vi "mk.vi"() -> ()   [LabVIEW 2016]
uses:
  <vilib>/Utility/file.llb/Write Delimited Spreadsheet (DBL).vi
panel:
  in  "Boolean 2":bool
  out "midiendo histeresis":bool
  in  "Boolean":bool
  in  "Lecturas":i32=5 min=1
  out "upset multimetro":dbl
  out "upset lockin":dbl
  out "division":cluster{"array":dbl[], "array":dbl[]}(graph)
  out "multimetro":cluster{"array":dbl[], "array":dbl[]}(graph)
  in  "Nombre (guardar como .txt)":path
  out "campo":dbl
  in  "paso":dbl
  in  "final":dbl
  in  "inicio":dbl
  out "Lock_In":cluster{"array":dbl[], "array":dbl[]}(graph)
  # "normal"
  # "histeresis"
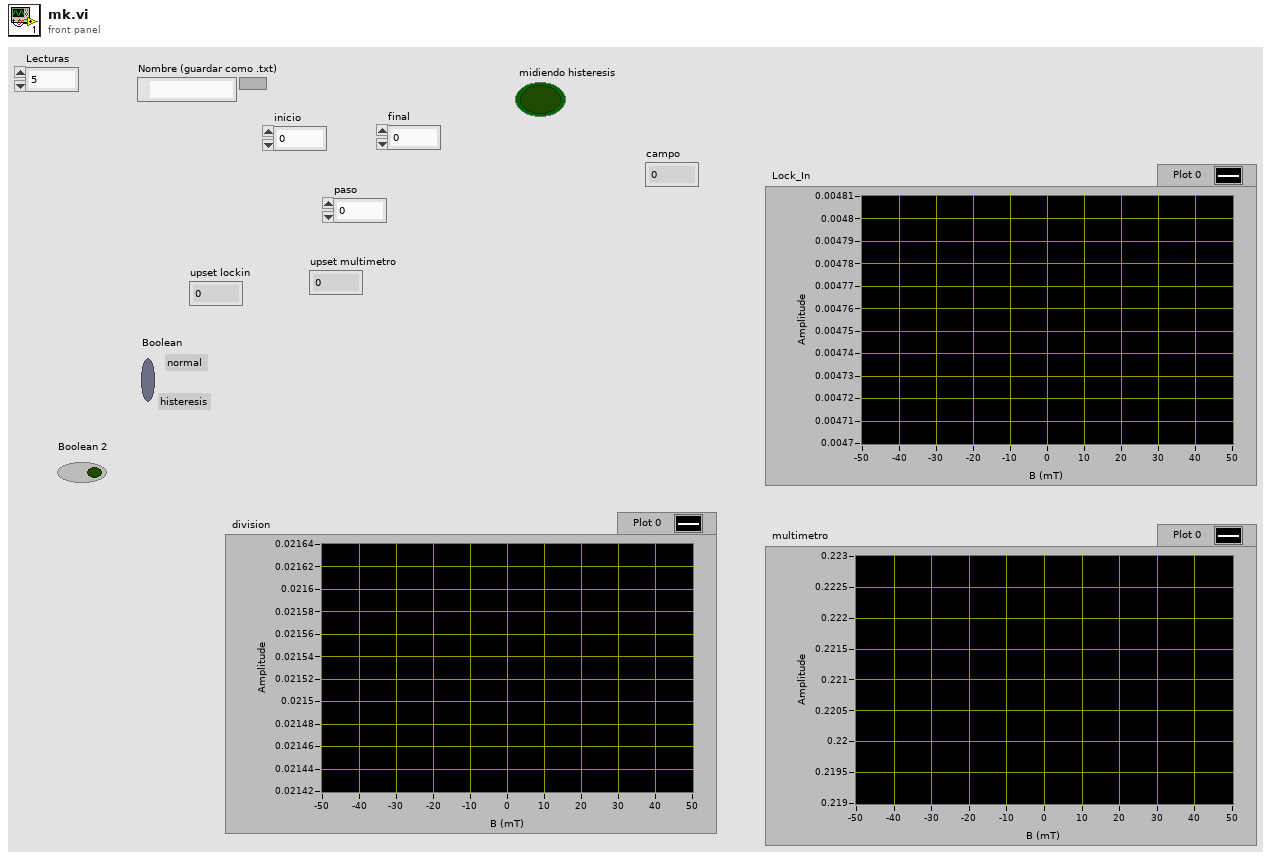
[diagram p1: front panel]
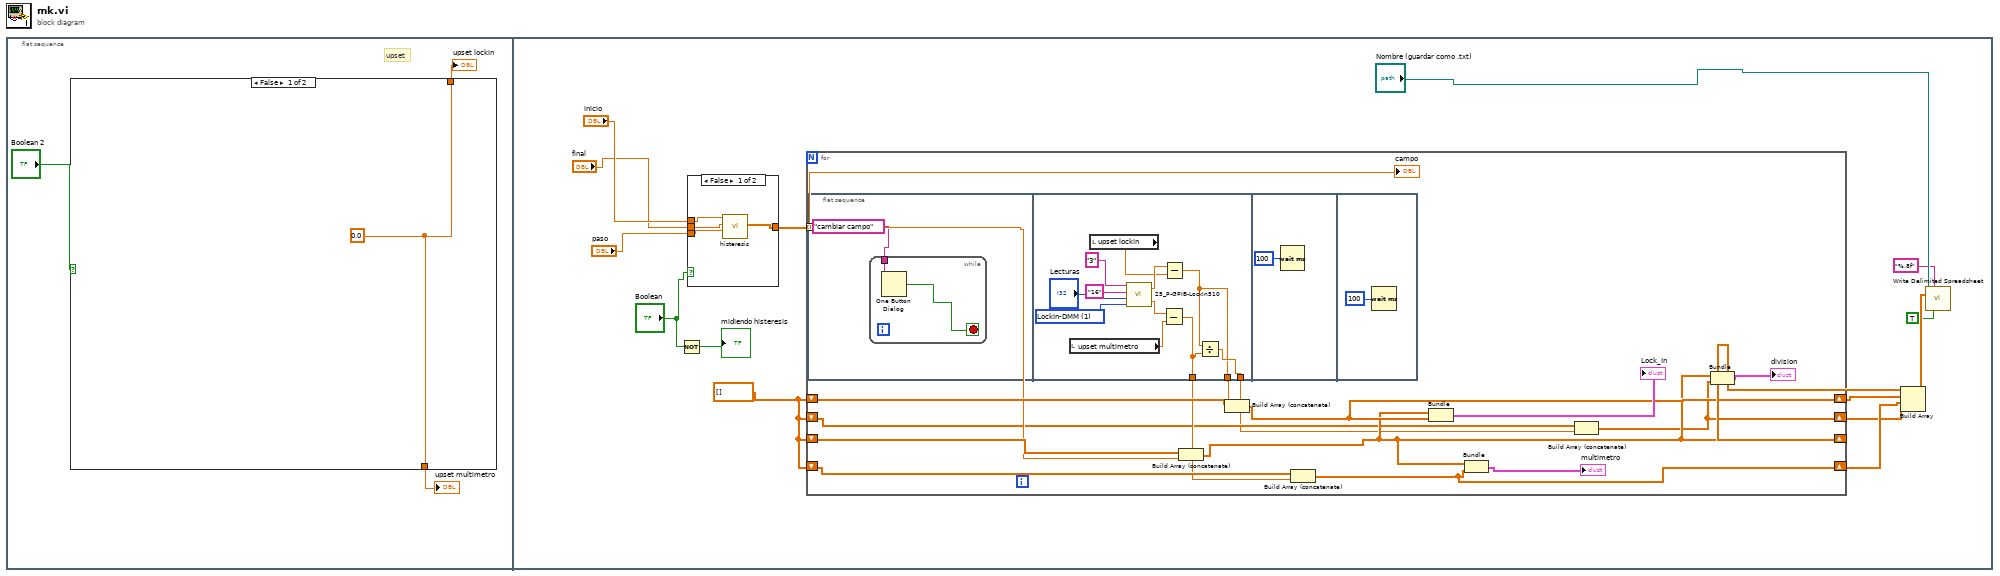
[diagram p0: block diagram]
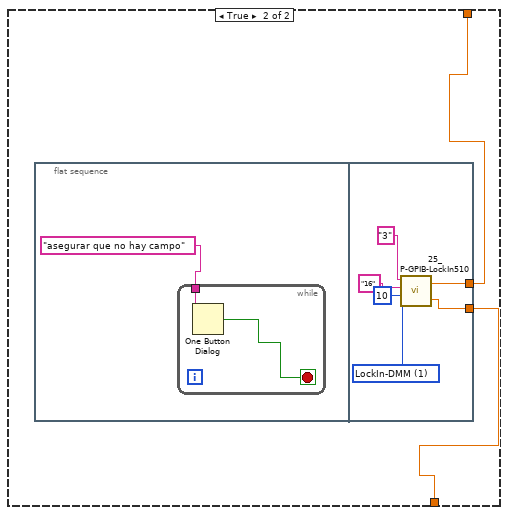
[diagram p2: hidden frame]
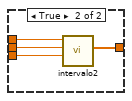
[diagram p3: hidden frame]
diagram:
  n1 = flat-sequence {
    frame #0 {
      # "upset"
      n2 = case shown="False" "Boolean 2" {
        tunnel: [w4 w6] -> w2
        tunnel: [w4 w5] -> w1
        frame False {
          w4 = 0.0
        }
        frame True {
          n3 = flat-sequence {
            tunnel: [w12] -> w6
            tunnel: [w11] -> w5
            frame #0 {
              n4 = while {
                tunnel: "asegurar que no hay campo" ("message") -> [w8]
                stop <- w9 stop-if-true
                n5 = One Button Dialog(message=w8) -> (true=w9:bool)  [unwired: 1 in]
              }
            }
            frame #1 {
              w13 = u16 1 items=["LockIn", "LockIn-DMM"] ("Tipo")
              n6 = call "25_P-GPIB-LockIn510.vi"("Tipo"=w13, "Lecturas"=10, "P-DMM"="16", "P-LockIn"="3") -> ("DMM"=w11:dbl, "LockIn"=w12:dbl)
            }
          }
        }
      }
      "upset lockin" <- w2
      "upset multimetro" <- w1
    }
    frame #1 {
      w19 = dbl[] []
      n7 = Not(x="Boolean") -> (.not. x?=→"midiendo histeresis":bool)
      n8 = case shown="False" "Boolean" {
        tunnel: "inicio" -> [w33 w38]
        tunnel: "final" -> [w32 w37]
        tunnel: "paso" -> [w31 w36]
        tunnel: [w34 w35] -> w27
        frame False {
          n9 = call "histeresis.vi"("paso"=w31, "fin"=w32, "inicio"=w33) -> ("Array"=w34:dbl[])  [unwired: 8 in]
        }
        frame True {
          n10 = call "intervalo2.vi"("incremento"=w36, "fin"=w37, "inicio"=w38) -> ("Array"=w35:dbl[])  [unwired: 8 in]
        }
      }
      n11 = for {
        tunnel: w27 -> [w49] mode=indexing
        shift-right: [w47] -> w21
        shift-left: w19 -> [w52]
        shift-right: [w43] -> w25
        shift-left: w19 -> [w51]
        shift-right: [w45] -> w20
        shift-left: w19 -> [w46]
        shift-right: [w39] -> w18
        shift-left: w19 -> [w41]
        n12 = flat-sequence {
          tunnel: [w62] -> w53
          tunnel: [w59] -> w42
          tunnel: [w63] -> w40
          frame #0 {
            n13 = while {
              tunnel: "cambiar campo" ("message") -> [w55]
              stop <- w56 stop-if-true
              n14 = One Button Dialog(message=w55) -> (true=w56:bool)  [unwired: 1 in]
            }
          }
          frame #1 {
            w64 = u16 1 items=["LockIn", "LockIn-DMM"] ("Tipo")
            n15 = local read "upset multimetro"() -> (w57:dbl)
            n16 = local read "upset lockin"() -> (w60:dbl)
            n17 = call "25_P-GPIB-LockIn510.vi"("Tipo"=w64, "Lecturas"="Lecturas", "P-DMM"="16", "P-LockIn"="3") -> ("DMM"=w58:dbl, "LockIn"=w61:dbl)
            n18 = Subtract(x=w58, y=w57) -> (x-y=w59:dbl)
            n19 = Subtract(x=w61, y=w60) -> (x-y=w62:dbl)
            n20 = Divide(x=w62, y=w59) -> (x/y=w63:dbl)
          }
          frame #2 {
            n21 = Wait (ms)(milliseconds to wait=u32 100) -> ()  [unwired: 1 out]
          }
          frame #3 {
            n22 = Wait (ms)(milliseconds to wait=u32 100) -> ()  [unwired: 1 out]
          }
        }
        n23 = Build Array (concatenate)(w51, w49) -> (w43:dbl[])
        n24 = Build Array (concatenate)(w52, w53) -> (w47:dbl[])
        n25 = Build Array (concatenate)(w46, w42) -> (w45:dbl[])
        n26 = Bundle(w43, w47) -> (→"Lock_In":cluster{dbl[], dbl[]})  [unwired: 1 in]
        n27 = Bundle(w43, w45) -> (→"multimetro":cluster{dbl[], dbl[]})  [unwired: 1 in]
        n28 = Build Array (concatenate)(w41, w40) -> (w39:dbl[])
        n29 = Bundle(w43, w39) -> (→"division":cluster{dbl[], dbl[]})  [unwired: 1 in]
        "campo" <- w49
      }
      n30 = Build Array(w25, w21, w20, w18) -> (w24:dbl[][])
      n31 = call-poly <vilib>:"Write Delimited Spreadsheet.vi"("file path (dialog if empty)"="Nombre (guardar como .txt)", "format (%.3f)"="%.8f", "2D data"=w24, "transpose? (no:F)"=TRUE) -> ()  [unwired: 10 in, 2 out]
    }
  }
